vi "pp_writeStimulus.vi"(0 "Current/Cued Trial":T2={"Trial Code"=1, "Trial Type"=enum."GO", "Trial Weight"=0, "Stim Type"=enum."FM Sweep", "Stim Dur (s)"=2.0, "Stim P1"=4.0, "Stim P2"=0.0} {"Stim P2" min=0.0; "Trial Weight" step=1; "Stim P1" min=0.0; "Stim Dur (s)" min=0.0; "Trial Code" min=1 step=1}, 2 "DAQmx Analog Out In":refnum<k21>, 3 "DAQmx Digital Out 1 In":refnum<k21>, 4 "DAQmx Digital Out 2 In":refnum<k21>, 5 "Error In":errorcluster, 8 "Waveform Properties":T1={"Fs (Hz)"=20000.0, "Amplitude (V)"=5.0, "Ramp (s)"=0.005, "Duration (s)"=0.25} {"Ramp (s)" min=0.0; "Fs (Hz)" min=0.0}) -> (15 "Waveform Out":waveform(dbl)={"t0"=timestamp(0 s since 1904-01-01), "dt"=5e-05, "Y"=array[2000 elements]}, 16 "DAQmx Analog Out Out":refnum<k21>, 17 "DAQmx Digital Out 1 Out":refnum<k21>, 18 "DAQmx Digital Out 2 Out":refnum<k21>, 19 "Error Out":errorcluster)   [LabVIEW 2013]
uses:
  <vilib>/DAQmx/write.llb/DAQmx Write (Analog DBL 1Chan 1Samp).vi
  <vilib>/DAQmx/write.llb/DAQmx Write (Digital U8 1Chan 1Samp).vi
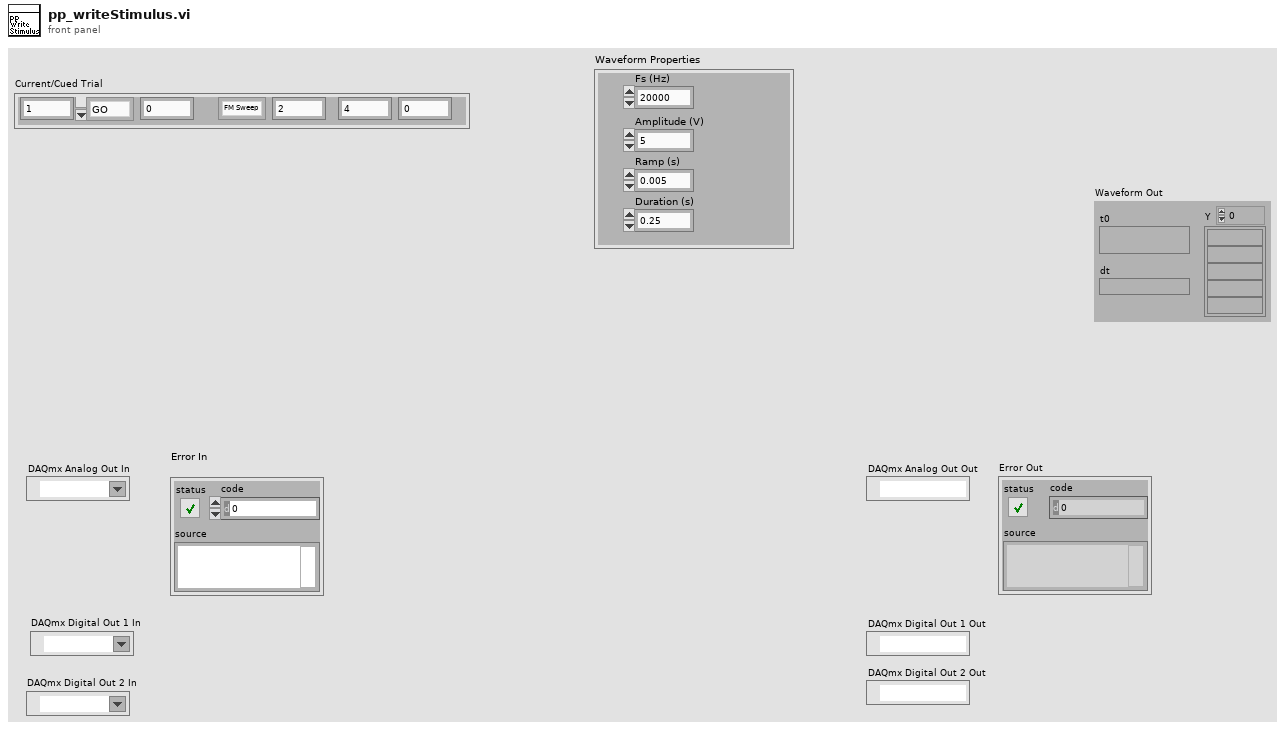
[diagram p1: front panel]
types:
  T1 = cluster{"Fs (Hz)":dbl, "Amplitude (V)":dbl, "Ramp (s)":dbl, "Duration (s)":dbl}
  T2 = cluster{"Trial Code":u16, "Trial Type":enum16{"OFF", "GO", "NOGO", "TEST"}, "Trial Weight":u32, "Stim Type":enum16{"Pure Tone", "FM Sweep"}, "Stim Dur (s)":dbl, "Stim P1":dbl, "Stim P2":dbl}
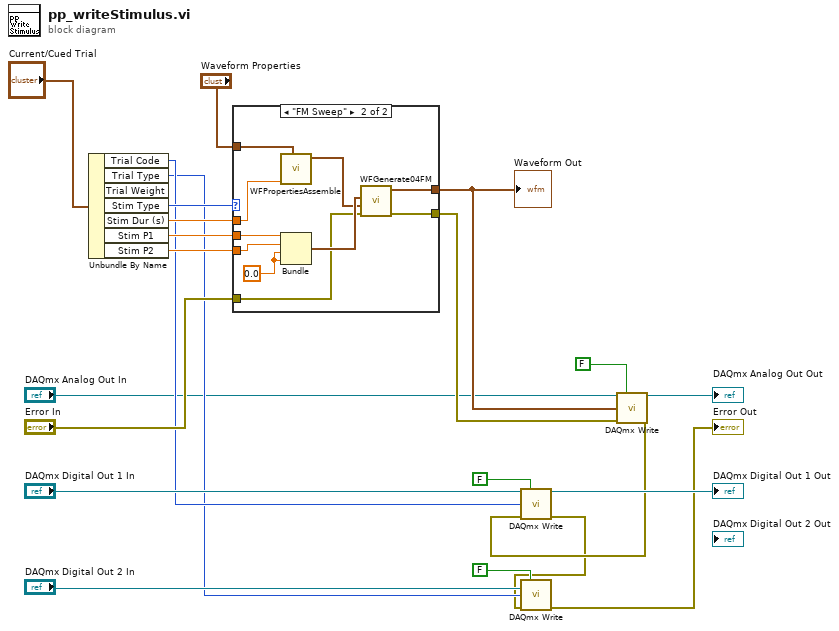
[diagram p0: block diagram]
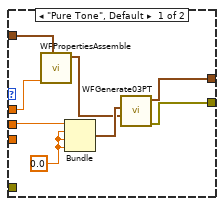
[diagram p2: hidden frame]
diagram:
  n1 = Unbundle By Name("Current/Cued Trial") -> ("Trial Code"=w10:u16, "Trial Type"=w7:enum16{"OFF", "GO", "NOGO", "TEST"}, "Stim Type"=w16:enum16{"Pure Tone", "FM Sweep"}, "Stim Dur (s)"=w12:dbl, "Stim P1"=w14:dbl, "Stim P2"=w13:dbl)  [unwired: 1 out]
  n2 = case shown="\"FM Sweep\"" w16 {
    tunnel: "Waveform Properties" -> [w30 w36]
    tunnel: w14 -> [w25 w40]
    tunnel: w13 -> [_ w39]
    tunnel: w12 -> [w29 w34]
    tunnel: [w23 w33] -> w3
    tunnel: "Error In" -> [_ w32]
    tunnel: [w24 w31] -> w2
    frame "Pure Tone", Default {
      w26 = 0.0
      n3 = call "WFPropertiesAssemble.vi"("Waveform Properties Previous"=w30, "Duration (s)"=w29) -> ("Waveform Properties"=w27:T1)  [unwired: 9 in]
      n4 = Bundle("Stim P1"=w25, w26, w26, w26) -> (w28:cluster{"Stim P1":dbl, dbl, dbl, dbl})  [unwired: 1 in]
      n5 = call "WFGenerate03PT.vi"("Waveform Properties"=w27, "Waveform Parameters"=w28) -> ("error out"=w24:errorcluster, "Waveform Out"=w23:waveform(dbl))  [unwired: 8 in]
    }
    frame "FM Sweep" {
      w37 = 0.0
      n6 = call "WFPropertiesAssemble.vi"("Waveform Properties Previous"=w36, "Duration (s)"=w34) -> ("Waveform Properties"=w35:T1)  [unwired: 9 in]
      n7 = Bundle("Stim P1"=w40, "Stim P2"=w39, w37, w37) -> (w38:cluster{"Stim P1":dbl, "Stim P2":dbl, dbl, dbl})  [unwired: 1 in]
      n8 = call "WFGenerate04FM.vi"("error in (no error)"=w32, "Waveform Properties"=w35, "Waveform Parameters"=w38) -> ("error out"=w31:errorcluster, "Waveform Out"=w33:waveform(dbl))  [unwired: 7 in]
    }
  }
  "Waveform Out" <- w3
  n9 = call-poly <vilib>:"DAQmx Write.vi"("task/channels in"="DAQmx Analog Out In", "auto start"=FALSE, "data"=w3, "error in"=w2) -> ("task out"=→"DAQmx Analog Out Out":refnum<k21>, "error out"=w6:errorcluster)  [unwired: 9 in, 1 out]
  n10 = call-poly <vilib>:"DAQmx Write.vi"("task/channels in"="DAQmx Digital Out 1 In", "auto start"=FALSE, "data"=w10, "error in"=w6) -> ("task out"=→"DAQmx Digital Out 1 Out":refnum<k21>, "error out"=w5:errorcluster)  [unwired: 9 in, 1 out]
  n11 = call-poly <vilib>:"DAQmx Write.vi"("task/channels in"="DAQmx Digital Out 2 In", "auto start"=FALSE, "data"=w7, "error in"=w5) -> ("error out"=→"Error Out":errorcluster)  [unwired: 9 in, 2 out]
